vi "XIPIN_Multiplier_11_2.vi"   [LabVIEW 2017]
doc: "Multiplication is a fundamental DSP operation. This core allows parallel and constant-coefficient multipliers to be generated. The user can specify if dedicated hardware multipliers, slice logic or a combination of resources should be utilized.\n------------------------------------\n<b>Need License</b> : No"
uses:
  <vilib>/rvi/XilinxIP/XIPIN_XNode/niFpgaXIPIN.xnode
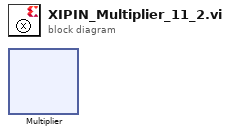
[diagram p0: block diagram]
diagram:
  n1 = xnode ("Multiplier")() -> ()
